vi "get unique channel name.vi"(8 "error in":errorcluster, 9 "prefix":string, 10 "scale name":string, 11 "channels":refnum<class "TBM channel.lvclass">[](array[class])) -> (0 "error out":errorcluster, 3 "name":string)   [LabVIEW 2013, in "Scaling configuration.lvclass"]
uses:
  Scaling configuration.lvclass
  <vilib>/NI/Tag Bus Module Framework/channel/TBM channel.lvclass
  <vilib>/NI/Tag Bus/tag/tag descriptor.lvclass/tag descriptor.ctl
  <vilib>/NI/Tag Bus/tag/tag descriptor.lvclass
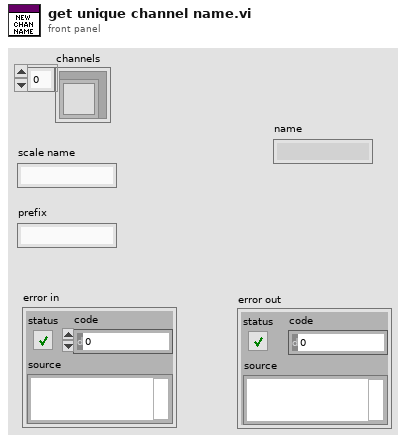
[diagram p1: front panel]
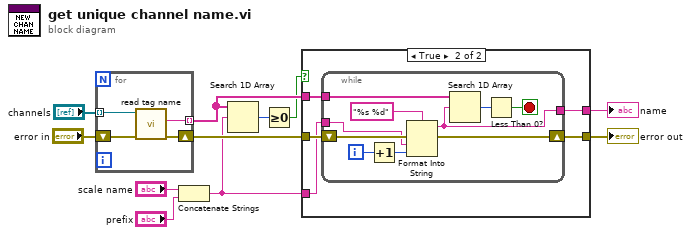
[diagram p0: block diagram]
diagram:
  n1 = for {
    tunnel: "channels" -> [w15] mode=indexing
    tunnel: [w14] -> w4 mode=indexing
    shift-right: [w13] -> w7
    shift-left: "error in" -> [w12]
    n2 = call <vilib>:"read tag name.vi"("error in"=w12, "system tag in"=w15) -> ("error out"=w13:errorcluster, "name"=w14:string)  [unwired: 7 in, 1 out]
  }
  n3 = Concatenate Strings("scale name", "prefix") -> (w3:string)
  n4 = Search 1D Array(1D array=w4, element=w3) -> (index of element=w2:i32)  [unwired: 1 in]
  n5 = Greater Or Equal To 0?(x=w2) -> (x >= 0?=w1:bool)
  n6 = case shown="True" w1 {
    tunnel: w3 -> [w17 w18]
    tunnel: [w17 w22] -> w8
    tunnel: w4 -> [_ w19]
    tunnel: w7 -> [w16 w21]
    tunnel: [w16 w20] -> w6
    frame False {
    }
    frame True {
      n7 = while {
        tunnel: [w27] -> w22
        shift-right: [w25] -> w20
        shift-left: w21 -> [w26]
        tunnel: w19 -> [w24]
        tunnel: w18 -> [w23]
        i -> [w31]
        stop <- w28 stop-if-true
        n8 = Increment(x=w31) -> (x+1=w30:i32)
        n9 = Format Into String(format string="%s %d", error in=w26, w23, w30) -> (resulting string=w27:string, error out=w25:errorcluster)  [unwired: 1 in]
        n10 = Search 1D Array(1D array=w24, element=w27) -> (index of element=w29:i32)  [unwired: 1 in]
        n11 = Less Than 0?(x=w29) -> (x < 0?=w28:bool)
      }
    }
  }
  "name" <- w8
  "error out" <- w6
